vi "Velmex cfg zero encoder.vi"(8 "error in (no error)":errorcluster {"code" format="%.0x"}, 9 "Simulation":T1, 10 "Channel parsed command info":T2, 11 "input cluster":refnum<class "VelmexStage.lvclass">) -> (0 "error out":errorcluster, 2 "new commands":string, 3 "output cluster":refnum<class "VelmexStage.lvclass">)   [LabVIEW 2020, in "VelmexStage.lvclass"]
uses:
  VelmexStage.lvclass
  channel parsed cmd cluster.ctl
  OnOffTypeDef.ctl
  VelmexStage.lvclass/VelmexStage.ctl
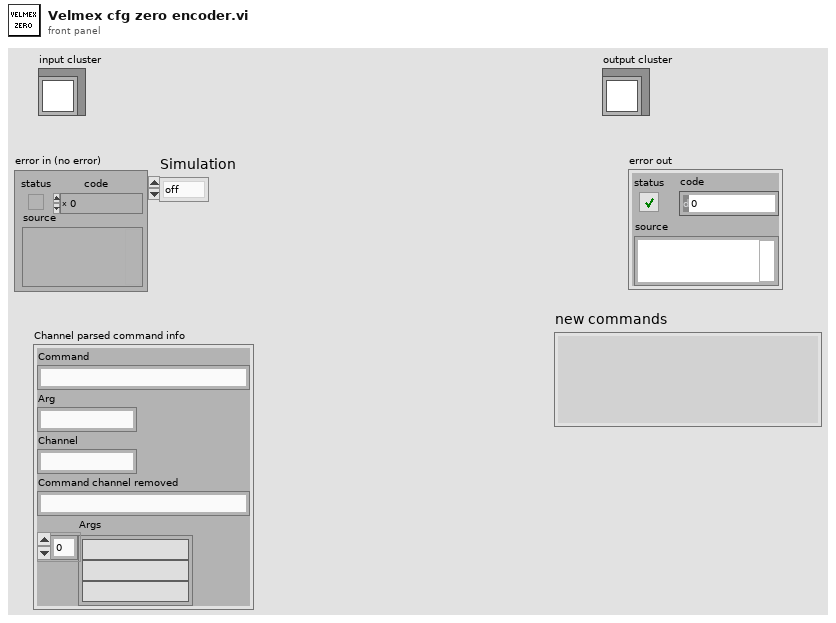
[diagram p1: front panel]
types:
  T1 = typedef "OnOffTypeDef.ctl" = enum16{"off", "on"}
  T2 = typedef "channel parsed cmd cluster.ctl" = cluster{"Command":string, "Arg":string, "Channel":string, "Command channel removed":string, "Args":string[]}
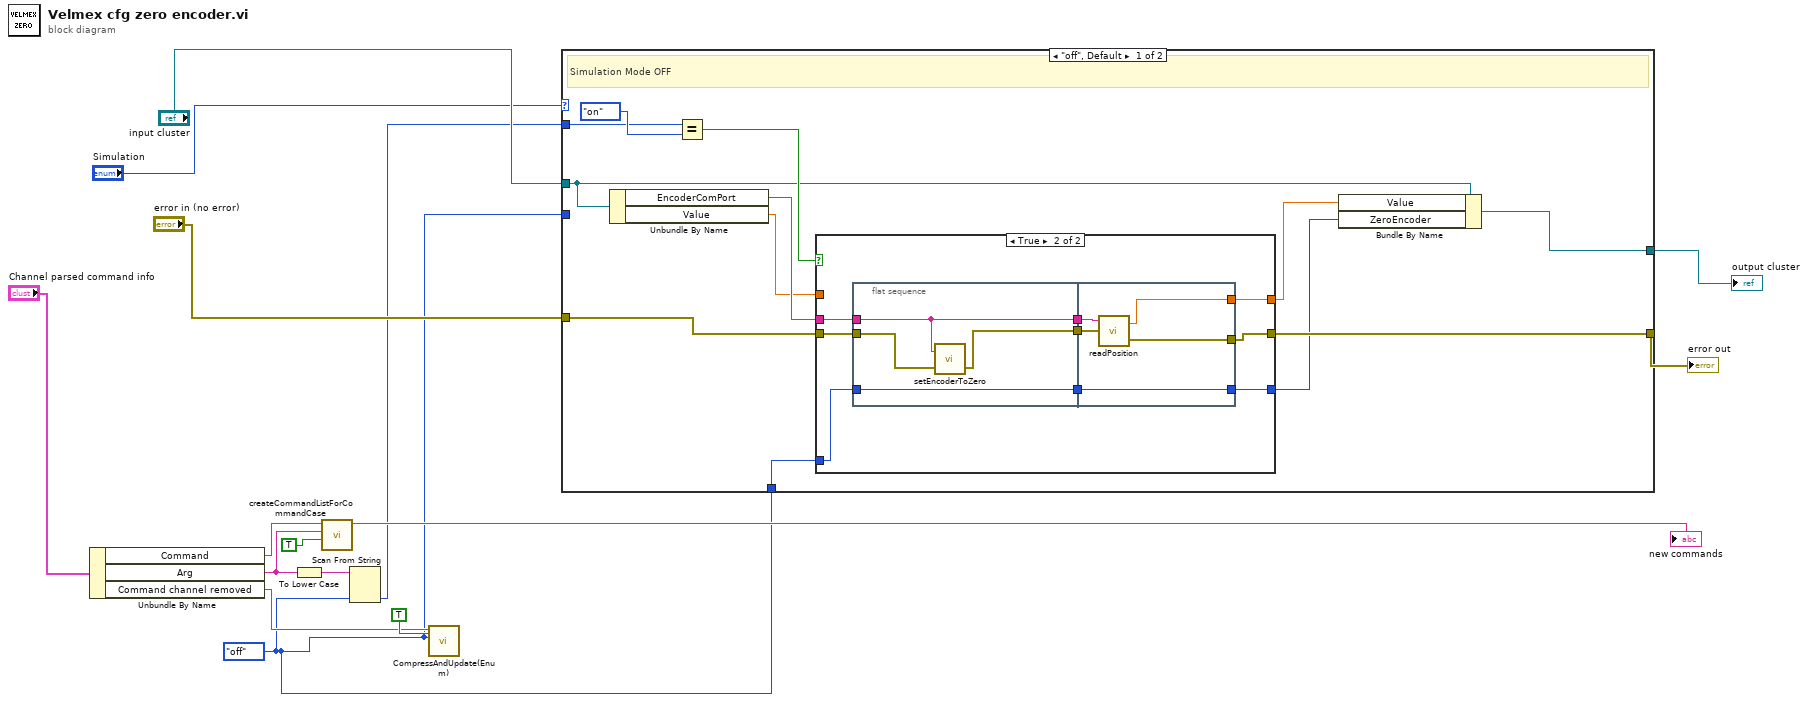
[diagram p0: block diagram]
diagram:
  w1 = enum16{"off", "on"}."off"
  n1 = Unbundle By Name("Channel parsed command info") -> ("Command"=w14:string, "Arg"=w5:string, "Command channel removed"=w3:string)
  n2 = To Lower Case(string=w5) -> (all lower case string=w6:string)
  n3 = call "createCommandListForCommandCase.vi"("immediate Check (only once)"=TRUE, "setvalue"=w5, "command"=w14) -> ("new commands"=→"new commands":string)  [unwired: 8 in]
  n4 = Scan From String(input string=w6, default 1=w1) -> (output 1=w4:enum16{"off", "on"})  [unwired: 3 in, 3 out]
  n5 = call "CompressAndUpdate(Enum).vi"("force CVT update (false)"=TRUE ("force CVT update"), "enum variant"=w1, "command or variable name"=w3) -> ()  [unwired: 8 in, 1 out]
  n6 = case shown="\"off\", Default" "Simulation" {
    tunnel: [w23 w49] -> w10
    tunnel: "input cluster" -> [w21 w50]
    tunnel: "error in (no error)" -> [w24 w49]
    tunnel: [w20 w50] -> w11
    tunnel: w4 -> [w26 _]
    tunnel: w1 -> [_ _]
    tunnel: w1 -> [w18 _]
    frame "off", Default {
      # "Simulation Mode OFF"
      n7 = Unbundle By Name(w21) -> ("EncoderComPort"=w19:string, "Value"=w16:dbl)
      n8 = Equal?(x=w26, y=enum16{"off", "on"}."on") -> (x = y?=w25:bool)
      n9 = case shown="True" w25 {
        tunnel: w24 -> [w30 w36]
        tunnel: [w30 w35] -> w23
        tunnel: w19 -> [_ w38]
        tunnel: [w28 w34] -> w22
        tunnel: w18 -> [w29 w33]
        tunnel: [w29 w31] -> w17
        tunnel: w16 -> [w28 _]
        frame False {
        }
        frame True {
          n10 = flat-sequence {
            tunnel: [w42] -> w39
            tunnel: w38 -> [w42]
            tunnel: [w40] -> w37
            tunnel: w36 -> [w41]
            tunnel: w33 -> [w43]
            tunnel: [w43] -> w32
            tunnel: w39 -> [w48]
            tunnel: w37 -> [w47]
            tunnel: [w46] -> w35
            tunnel: [w45] -> w34
            tunnel: [w44] -> w31
            tunnel: w32 -> [w44]
            frame #0 {
              n11 = call "setEncoderToZero.vi"("error in (no error)"=w41, "VISA resource name"=w42) -> ("error out"=w40:errorcluster)  [unwired: 1 out]
            }
            frame #1 {
              n12 = call "readPosition.vi"("error in (no error)"=w47, "VISA resource name"=w48) -> ("error out"=w46:errorcluster, "position"=w45:dbl)  [unwired: 1 out]
            }
          }
        }
      }
      n13 = Bundle By Name(cluster=w21, "Value"=w22, "ZeroEncoder"=w17) -> (w20:refnum<class "VelmexStage.lvclass">)
    }
    frame "on" {
      # "Simulation Mode ON"
    }
  }
  "output cluster" <- w11
  "error out" <- w10
